vi "FPGA_Top_Level_cRIO_Main.vi"() -> ()   [LabVIEW 2011]
uses:
  Controls/FPGA SPI_Cmd.ctl
  Controls/FPGA SPI_Arb Loop State.ctl
  <vilib>/rvi/eio/common/nirviEmuTemplateMethod_errors.vi
  Code/FPGA SPI_Globals.vi
  <vilib>/rvi/FIFO/Fifo_Resource/nirvififoEmulationSetSize.vi
  <vilib>/rvi/DataTransferAndStorage/Container/Common/niFpgaContainerGetUniqueNameForEmu.vi
  <vilib>/eio/EIONode/EIONode.xnode
  <vilib>/rvi/DataTransferAndStorage/Container/XNode/niFpgaContainer.xnode
  <vilib>/rvi/FIFO/Fifo_Resource/nirvififoEmulationWrite.vi
  <vilib>/rvi/FIFO/Fifo_Resource/nirvififoEmulationRead.vi
panel:
  in  "SPI_Clock Divider":u32=20
  in  "SPI_CS Active State":bool caption="SPI_CS\nActive State"
  in  "SPI_CPOL":bool
  in  "SPI_CPHA":bool
  in  "SPI_CS":u8=1 format="%08b"
  in  "SPI_Total Bits":u16=8
  in  "SPI_Total Bytes":u16=1
  in  "SPI_Start":bool
  in  "SPI_Cmd":T1=enum."Configure"
  in  "SPI_Ack Read":bool
  out "SPI_Read Data":u8
  out "SPI_Read Flag":bool
  in  "SPI_Write Flag":bool
  in  "SPI_Write Data":u8
  in  "SPI_Port":u8
  # "Control"
  # "SPI Configuration Parameters"
  # "Command Type"
  # "Host Data Transfer"
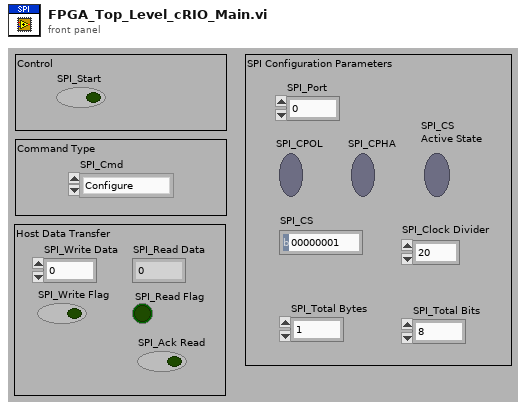
[diagram p1: front panel]
types:
  T1 = typedef "FPGA SPI_Cmd.ctl" = enum8{"Idle", "Write/Read SPI", "Configure"}
  T2 = cluster{"SCLK":refnum<k21>, "CS_1":refnum<k21>, "MOSI":refnum<k21>, "MISO":refnum<k21>, "CS_2":refnum<k21>}
  T3 = typedef "FPGA SPI_Arb Loop State.ctl" = enum8{"Idle", "Init", "Write", "Start", "Read", "Wait Until Done"}
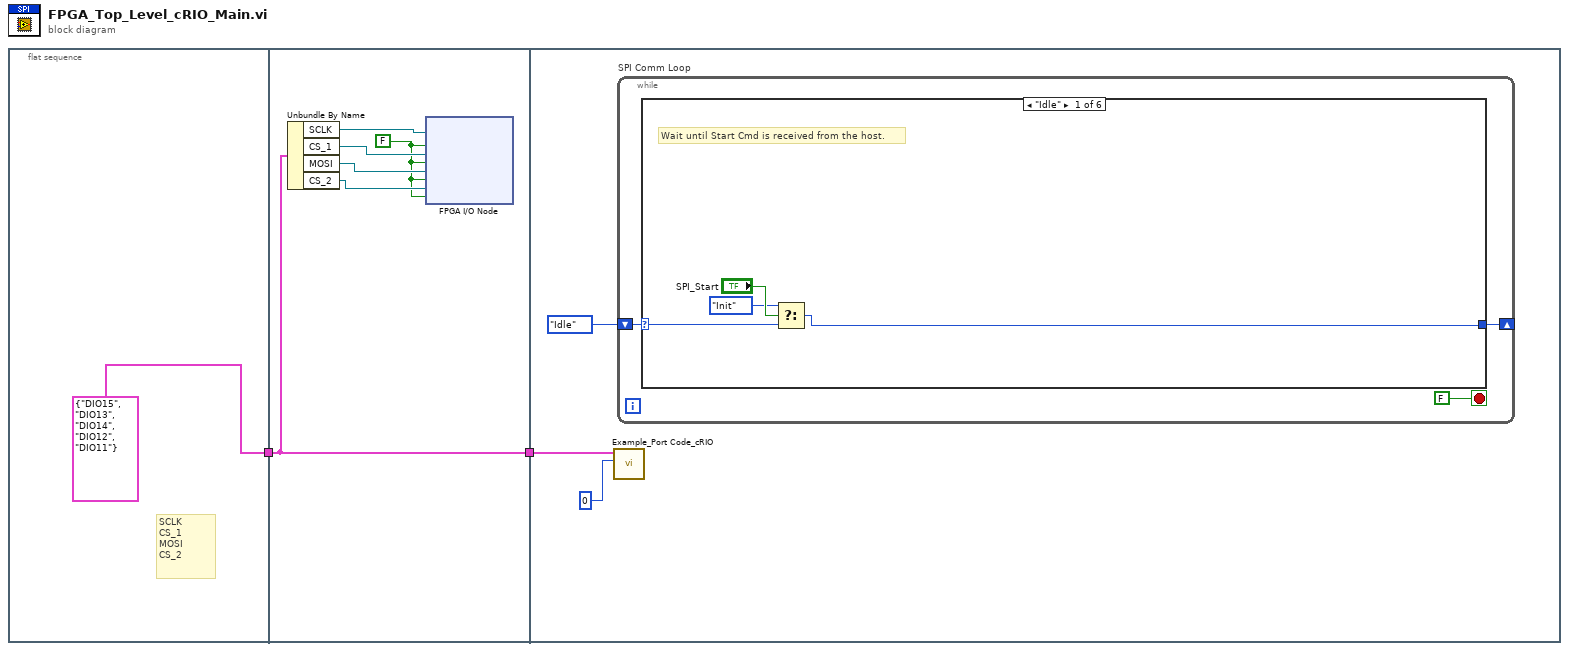
[diagram p0: block diagram]
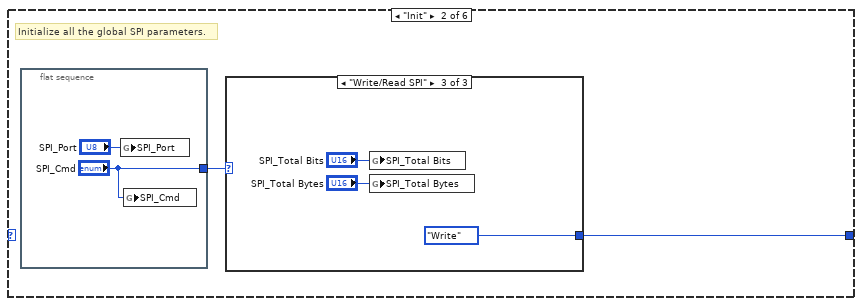
[diagram p2: hidden frame]
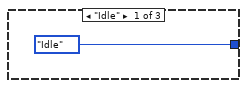
[diagram p3: hidden frame]
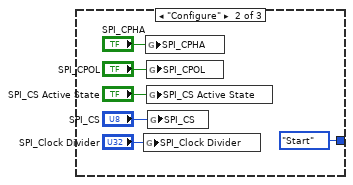
[diagram p4: hidden frame]
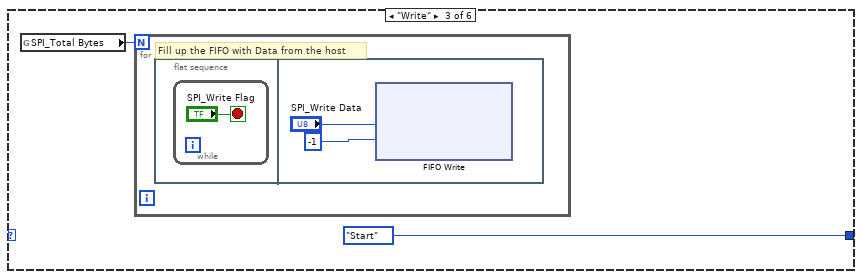
[diagram p5: hidden frame]
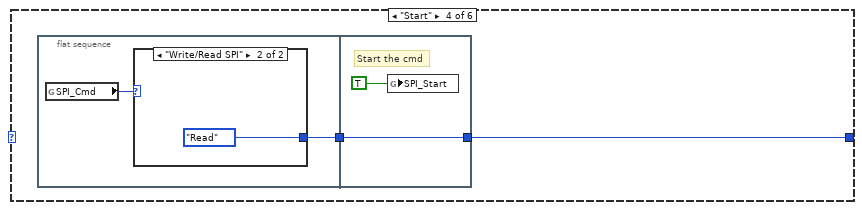
[diagram p6: hidden frame]
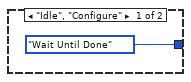
[diagram p7: hidden frame]
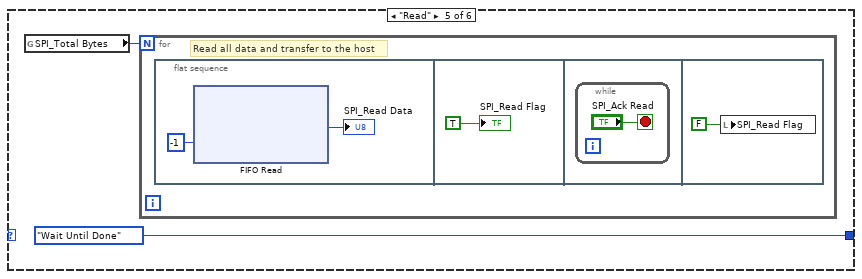
[diagram p8: hidden frame]
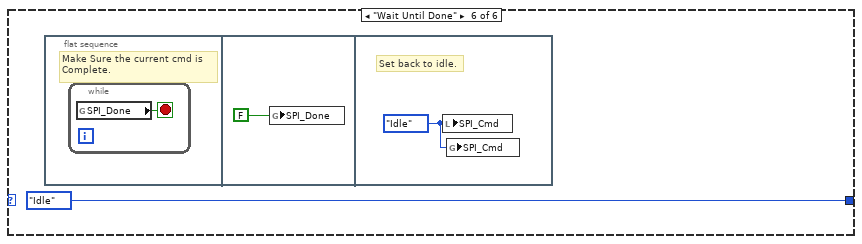
[diagram p9: hidden frame]
diagram:
  n1 = flat-sequence {
    tunnel: [T2 {"SCLK"="DIO15", "CS_1"="DIO13", "MOSI"="DIO14", "MISO"="DIO12", "CS_2"="DIO11"} ("FPGA I/O")] -> w2
    tunnel: w2 -> [w4]
    tunnel: [w4] -> w1
    tunnel: w1 -> [w10]
    frame #0 {
      # "SCLK\nCS_1\nMOSI\nCS_2"
    }
    frame #1 {
      w6 = FALSE ("I/O Item")
      n2 = Unbundle By Name(w4) -> ("SCLK"=w5:refnum<k21>, "CS_1"=w9:refnum<k21>, "MOSI"=w8:refnum<k21>, "CS_2"=w7:refnum<k21>)
      n3 = xnode "FPGA I/O Node"("I/O Item"=w6, "FPGA I/O In"=w5, "I/O Item"=w6, "FPGA I/O In"=w9, "I/O Item"=w6, "FPGA I/O In"=w8, "I/O Item"=w6, "FPGA I/O In"=w7) -> ()  [unwired: 4 out]
    }
    frame #2 {
      n4 = call "Example_Port Code_cRIO.vi"("Port"=i8 0, "FPGA I/O"=w10) -> ()  [unwired: 10 out]
      n5 = while "SPI Comm Loop" {
        shift-right: [w14] -> _
        shift-left: FPGA_SPI_Arb_Loop_State."Idle" ("Action") -> [w13]
        stop <- FALSE stop-if-true
        n6 = case shown="\"Idle\"" w13 {
          selector: w13 -> [w18 _ _ _ _ _]
          tunnel: [w16 w20 FPGA_SPI_Arb_Loop_State."Start" ("Action") w40 FPGA_SPI_Arb_Loop_State."Wait Until Done" ("Action") FPGA_SPI_Arb_Loop_State."Idle" ("Action")] -> w14
          frame "Idle" {
            # "Wait until Start Cmd is received from the host."
            n7 = Select(t=FPGA_SPI_Arb_Loop_State."Init" ("Action"), s="SPI_Start", f=w18) -> (s? t:f=w16:T3)
          }
          frame "Init" {
            # "Initialize all the global SPI parameters."
            n8 = flat-sequence {
              tunnel: ["SPI_Cmd"] -> w21
              frame #0 {
                n9 = global write "FPGA SPI_Globals.vi" "SPI_Port"("SPI_Port") -> ()
                n10 = global write "FPGA SPI_Globals.vi" "SPI_Cmd"("SPI_Cmd") -> ()
              }
            }
            n11 = case shown="\"Write/Read SPI\"" w21 {
              tunnel: [FPGA_SPI_Arb_Loop_State."Idle" ("Action") FPGA_SPI_Arb_Loop_State."Start" ("Action") FPGA_SPI_Arb_Loop_State."Write" ("Action")] -> w20
              frame "Idle" {
              }
              frame "Configure" {
                n12 = global write "FPGA SPI_Globals.vi" "SPI_Clock Divider"("SPI_Clock Divider") -> ()
                n13 = global write "FPGA SPI_Globals.vi" "SPI_CPHA"("SPI_CPHA") -> ()
                n14 = global write "FPGA SPI_Globals.vi" "SPI_CPOL"("SPI_CPOL") -> ()
                n15 = global write "FPGA SPI_Globals.vi" "SPI_CS Active State"("SPI_CS Active State") -> ()
                n16 = global write "FPGA SPI_Globals.vi" "SPI_CS"("SPI_CS") -> ()
              }
              frame "Write/Read SPI" {
                n17 = global write "FPGA SPI_Globals.vi" "SPI_Total Bits"("SPI_Total Bits") -> ()
                n18 = global write "FPGA SPI_Globals.vi" "SPI_Total Bytes"("SPI_Total Bytes") -> ()
              }
            }
          }
          frame "Write" {
            n19 = global read "FPGA SPI_Globals.vi" "SPI_Total Bytes"() -> (w35:u16)
            n20 = for {
              N: w35 -> [_]
              # "Fill up the FIFO with Data from the host"
              n21 = flat-sequence {
                frame #0 {
                  n22 = while {
                    stop <- "SPI_Write Flag" stop-if-true
                  }
                }
                frame #1 {
                  n23 = xnode ("FIFO Write")("Element"="SPI_Write Data", "Timeout"=-1) -> ()  [unwired: 1 in, 2 out]
                }
              }
            }
          }
          frame "Start" {
            n24 = flat-sequence {
              tunnel: [w41] -> w39
              tunnel: [w46] -> w40
              tunnel: w39 -> [w46]
              frame #0 {
                n25 = global read "FPGA SPI_Globals.vi" "SPI_Cmd"() -> (w42:T1)
                n26 = case shown="\"Write/Read SPI\"" w42 {
                  tunnel: [FPGA_SPI_Arb_Loop_State."Wait Until Done" ("Action") FPGA_SPI_Arb_Loop_State."Read" ("Action")] -> w41
                  frame "Idle", "Configure" {
                  }
                  frame "Write/Read SPI" {
                  }
                }
              }
              frame #1 {
                # "Start the cmd"
                n27 = global write "FPGA SPI_Globals.vi" "SPI_Start"(TRUE ("Write Flag")) -> ()
              }
            }
          }
          frame "Read" {
            n28 = global read "FPGA SPI_Globals.vi" "SPI_Total Bytes"() -> (w48:u16)
            n29 = for {
              N: w48 -> [_]
              # "Read all data and transfer to the host"
              n30 = flat-sequence {
                frame #0 {
                  n31 = xnode ("FIFO Read")("Timeout"=-1) -> ("Element"=→"SPI_Read Data":u8)  [unwired: 1 in, 2 out]
                }
                frame #1 {
                  "SPI_Read Flag" <- TRUE ("Read Flag")
                }
                frame #2 {
                  n32 = while {
                    stop <- "SPI_Ack Read" stop-if-true
                  }
                }
                frame #3 {
                  n33 = local write "SPI_Read Flag"(FALSE ("Read Flag")) -> ()
                }
              }
            }
          }
          frame "Wait Until Done" {
            n34 = flat-sequence {
              frame #0 {
                # "Make Sure the current cmd is\nComplete."
                n35 = while {
                  stop <- w55 stop-if-true
                  n36 = global read "FPGA SPI_Globals.vi" "SPI_Done"() -> (w55:bool)
                }
              }
              frame #1 {
                n37 = global write "FPGA SPI_Globals.vi" "SPI_Done"(FALSE ("Done")) -> ()
              }
              frame #2 {
                w57 = FPGA_SPI_Cmd."Idle" ("Type")
                # "Set back to idle."
                n38 = local write "SPI_Cmd"(w57) -> ()
                n39 = global write "FPGA SPI_Globals.vi" "SPI_Cmd"(w57) -> ()
              }
            }
          }
        }
      }
    }
  }
